vi "temporaryMessage.vi"(0 "milliseconds to wait":u32=1000, 1 "button name (\"OK\")":string, 2 "message":string="If you wait a little, I will disappear") -> ()   [LabVIEW 2021]
doc: "This is an example that shows how to have a message box pop up and exit with out having to press OK."
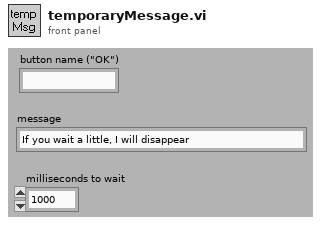
[diagram p1: front panel]
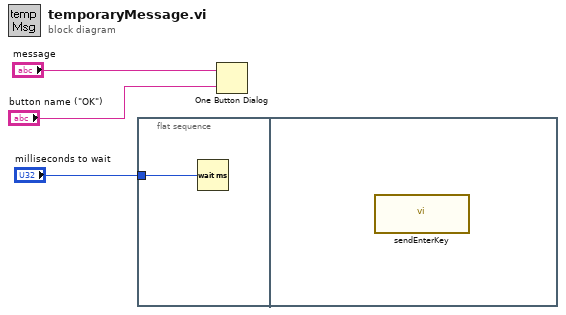
[diagram p0: block diagram]
diagram:
  n1 = flat-sequence {
    tunnel: "milliseconds to wait" -> [w4]
    frame #0 {
      n2 = Wait (ms)(milliseconds to wait=w4) -> ()  [unwired: 1 out]
    }
    frame #1 {
      n3 = call "sendEnterKey.vi"() -> ()  [unwired: 3 in]
    }
  }
  n4 = One Button Dialog(message="message", button name ("OK")="button name (\"OK\")") -> ()  [unwired: 1 out]
